vi "GEA2 Read and Update Message.vi"(0 "GEA2 Reference In":refnum<k24>, 1 "Update Information":string, 2 "Send Tries":u8=5 min=1 step=1, 3 "Read Timeout (ms)":u32=500, 5 "GEA Inputs":T2 {"Destination" format="%.0x"; "Source" format="%.0x"}, 7 "Read Command":u8 format="%.0x", 9 "Write Command":u8 format="%.0x", 11 "Error In":errorcluster, 12 "Expected Command":string=".*", 13 "Expected Data":string=".*", 14 "Send and Receive Tries":u8=5 min=1 step=1) -> (4 "GEA2 Reference Out":refnum<k24>, 6 "Updated Raw Data Out":string, 8 "Updated Converted Data Out":T1 {"CRC" format="%04x"; "Length" format="%02x"; "Command" format="%02x"; "Destination" format="%02x"; "Source" format="%02x"}, 15 "Error Out":errorcluster)   [LabVIEW 2019, in "GEA2_Toolkit.lvlib"]
doc: "This VI reads and updates GEA2 message based on the information provided in the Update information input. This VI only supports GEA2 commands that have a read and write command. The exact data read must be sendable to the write command. The update information should contain all of the bits that you wish to be updated in the ERD. Just specify the bits you want to update (ex. 0=1) and put whether or not you want them to be True (1) or False (0). You can specify a range of bits by using the - command in between two numbers (ex. 0-7=1 would change bits 0, 1, 2, 3, 4, 5, 6, 7 to true). The update information is converted to an array of strings by a comma delimiter. So, seperate your update information pieces by commas (Ex. if you wanted to make bits 0 and 10 false you could use the message: 0=0,10=0). Make sure you don't set the same bit twice or only the 2nd setting will ocurr (ex. 0=1,0=0 will only set bit 0 to false). If you were to write the following ERD data (00 01 02), byte 00 would be the byte 0 and contain bits 0-7, byte 01 would be byte 1 and contain bits 8-15, and byte 02 would be byte 2 and contain bits 16-23. For all bytes, the right-most bit is the first bit and the left-most bit is the last (Ex. For byte 00 being the hex value 0x01, bit 0 would be equal to 1 and would be the right-most bit (00000001)."
uses:
  library/GEA2_Toolkit.lvlib
  type defs/Data In.ctl
  D:/Common/LabVIEW GEA2 Toolkit/source/GEA3 DLL Source/GeaCommunication.dll
  source/GEA3 DLL Source/GeaCommunication.dll
  type defs/Source_Destination.ctl
  National Intruments Software/TestStand/GEA3/type defs/Data Out.ctl
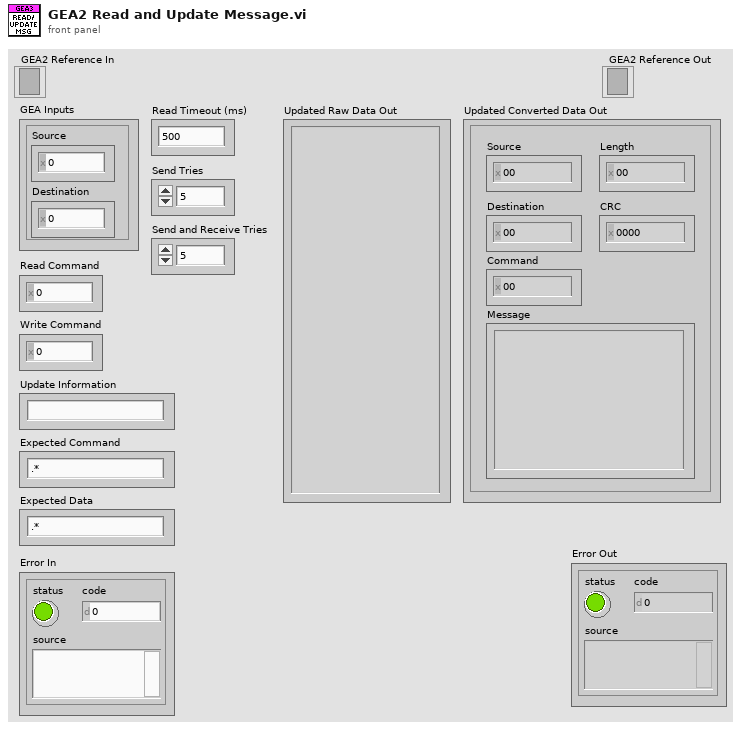
[diagram p1: front panel]
types:
  T1 = typedef "GEA2_Toolkit.lvlib/Data Out.ctl" = cluster{"Source":u8, "Destination":u8, "Command":u8, "Length":u8, "CRC":u16, "Message":string}
  T2 = typedef "GEA2_Toolkit.lvlib/Source_Destination.ctl" = cluster{"Source":u8, "Destination":u8}
  T3 = typedef "GEA2_Toolkit.lvlib/Data In.ctl" = cluster{"Source":u8, "Destination":u8, "Command":u8, "Message":string}
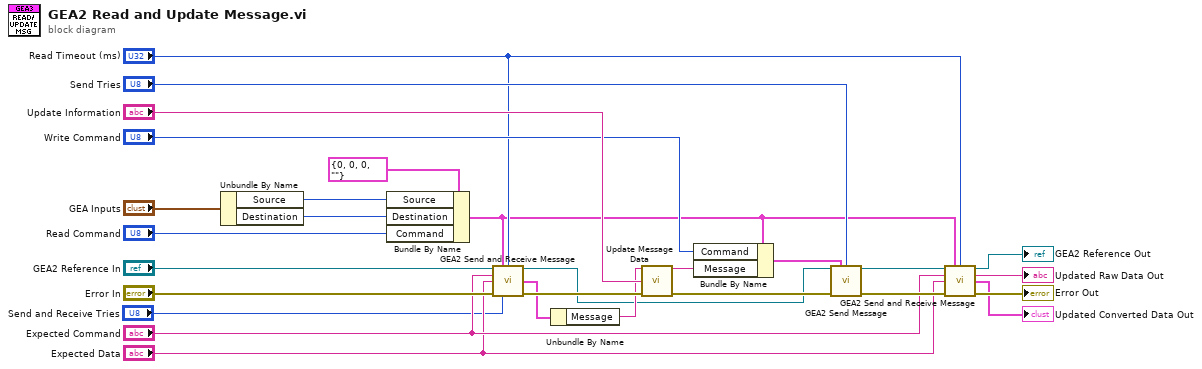
[diagram p0: block diagram]
diagram:
  n1 = Unbundle By Name("GEA Inputs") -> ("Source"=w17:u8, "Destination"=w16:u8)
  n2 = Bundle By Name(cluster=T3 {"Source"=0, "Destination"=0, "Command"=0, "Message"=""} ("Input Data"), "Source"=w17, "Destination"=w16, "Command"="Read Command") -> (w6:T3)
  n3 = call "GEA2 Send and Receive Message.vi"("GEA2 Reference In"="GEA2 Reference In", "Input Data"=w6, "Read Timeout (ms)"="Read Timeout (ms)", "Expected Command"="Expected Command", "Expected Data"="Expected Data", "Error In"="Error In", "# of Tries"="Send and Receive Tries") -> ("GEA2 Reference Out"=w21:refnum<k24>, "Converted Data Out"=w24:T1, "Error Out"=w27:errorcluster)  [unwired: 5 in, 1 out]
  n4 = Unbundle By Name(w24) -> ("Message"=w23:string)
  n5 = call "Update Message Data.vi"("Data In"=w23, "Update Information"="Update Information", "Error In"=w27) -> ("Data Out"=w13:string, "Error Out"=w22:errorcluster)  [unwired: 11 in]
  n6 = Bundle By Name(cluster=w6, "Command"="Write Command", "Message"=w13) -> (w12:T3)
  n7 = call "GEA2 Send Message.vi"("GEA2 Reference In"=w21, "Input Data"=w12, "# of Tries"="Send Tries", "Error In"=w22) -> ("GEA2 Reference Out"=w10:refnum<k24>, "Error Out"=w11:errorcluster)  [unwired: 10 in]
  n8 = call "GEA2 Send and Receive Message.vi"("GEA2 Reference In"=w10, "Input Data"=w6, "Read Timeout (ms)"="Read Timeout (ms)", "Expected Command"="Expected Command", "Expected Data"="Expected Data", "Error In"=w11) -> ("GEA2 Reference Out"=→"GEA2 Reference Out":refnum<k24>, "Raw Data Out"=→"Updated Raw Data Out":string, "Converted Data Out"=→"Updated Converted Data Out":T1, "Error Out"=→"Error Out":errorcluster)  [unwired: 6 in]
